vi "ReturnToNormalMode.vi"(8 "error in (no error)":errorcluster, 11 "connection info":T1) -> (0 "error out":errorcluster, 3 "connection info":T1)   [LabVIEW 2015, in "Diagnostics Host Automation API.lvlib"]
uses:
  Diagnostics Host Automation API.lvlib
  <vilib>/NI/STM/TCP/TCP Connection Info.ctl
  <vilib>/NI/STM/SubVIs/MetaDataElement.ctl
  <vilib>/NI/NIVS Addon Network Comm/Shared/NI VeriStand Addon Network Comm Shared.lvlib
  <vilib>/NI/STM/NI STM.lvlib
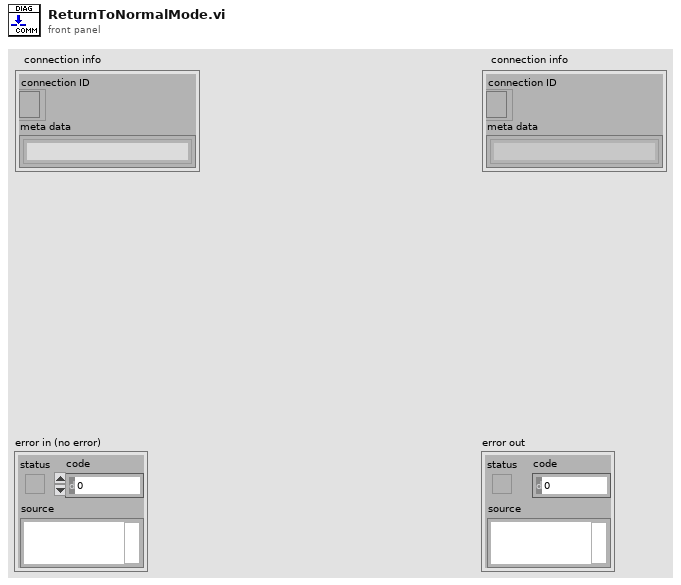
[diagram p1: front panel]
types:
  T1 = typedef "NI STM.lvlib/TCP Connection Info.ctl" = cluster{"connection ID":refnum<k5>, "meta data":T2[]}
  T2 = typedef "NI STM.lvlib/MetaDataElement.ctl" = string
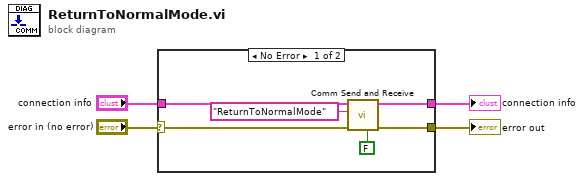
[diagram p0: block diagram]
diagram:
  n1 = case shown="No Error" "error in (no error)" {
    selector: "error in (no error)" -> [w6 w12]
    tunnel: "connection info" -> [w10 w11]
    tunnel: [w9 w11] -> w3
    tunnel: [w8 w12] -> w2
    frame No Error {
      n2 = call <vilib>:"Comm Send and Receive.vi"("Resp Required?"=FALSE, "error in (no error)"=w6, "Name"="ReturnToNormalMode", "connection info"=w10) -> ("error out"=w8:errorcluster, "connection info"=w9:T1)  [unwired: 4 in, 2 out]
    }
    frame Error {
    }
  }
  "connection info" <- w3
  "error out" <- w2
